vi "ziGetEventPWAWave.vi"(8 "Error In":errorcluster, 10 "PWAWaves In":T1[](array[typedef]) {"Frequency (Hz)" format="%#_6p"}, 11 "Handle In":T2 {"Handle" format="0x%08x"; "Conn" format="0x%08x"}) -> (0 "Error Out":errorcluster, 2 "PWAWaves Out":T1[](array[typedef]) {"Frequency (Hz)" format="%#_6p"}, 3 "Handle Out":T2 {"Handle" format="0x%08x"; "Conn" format="0x%08x"})   [LabVIEW 2009, in "Zurich Instruments LabOne.lvlib"]
uses:
  <instrlib>/Zurich Instruments LabOne/Zurich Instruments LabOne.lvlib
  <instrlib>/Zurich Instruments LabOne/Public/ziTypeHandle.ctl
  <instrlib>/Zurich Instruments LabOne/Public/Data/ziTypePWAWave.ctl
  <instrlib>/Zurich Instruments LabOne/Private/ziLV64.dll
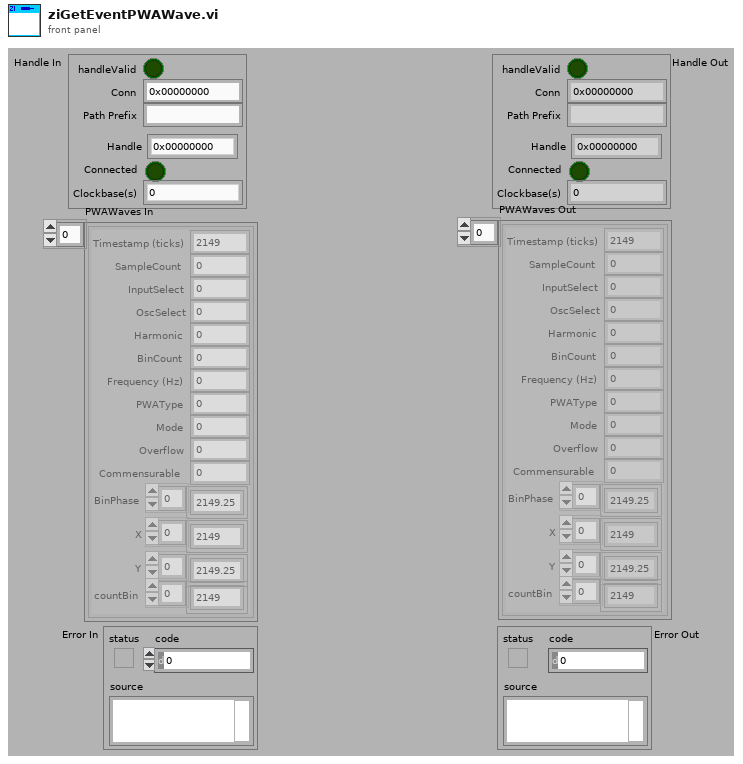
[diagram p1: front panel]
types:
  T1 = typedef "Zurich Instruments LabOne.lvlib/ziTypePWAWave.ctl" = cluster{"Timestamp (ticks)":u64, "SampleCount":u64, "InputSelect":i32, "OscSelect":i32, "Harmonic":i32, "BinCount":i32, "Frequency (Hz)":dbl, "PWAType":u8, "Mode":u8, "Overflow":u8, "Commensurable":u8, "BinPhase":dbl[], "X":dbl[], "Y":dbl[], "countBin":u32[]}
  T2 = typedef "Zurich Instruments LabOne.lvlib/ziTypeHandle.ctl" = cluster{"handleValid":bool, "Conn":u64, "Path Prefix":string, "Handle":u64, "Connected":bool, "Clockbase(s)":dbl}
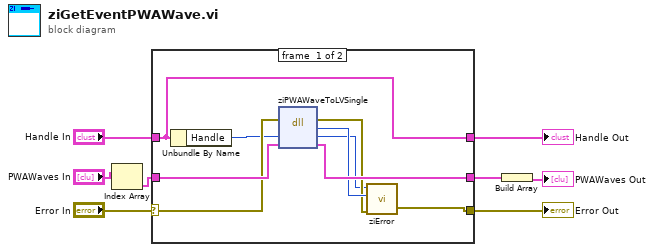
[diagram p0: block diagram]
diagram:
  n1 = Index Array(array="PWAWaves In") -> (element=w2:T1)  [unwired: 1 in]
  n2 = case shown="No Error" "Error In" {
    selector: "Error In" -> [w14 w18]
    tunnel: "Handle In" -> [w10 w20]
    tunnel: [w10 w20] -> w7
    tunnel: [w17 w18] -> w6
    tunnel: w2 -> [w16 w19]
    tunnel: [w15 w19] -> w4
    frame #0 {
      n3 = Unbundle By Name(w10) -> ("Handle"=w13:u64)
      n4 = dll-call lib="C:/Program Files/National Instruments/LabVIEW 2009/instr.lib/Zurich Instruments LabOne/Private/ziLV*.*" fn="ziPWAWaveToLVSingle"(error in=w14, "ziEventBuffer"=w13, "PWAWave"=w16) -> (error out=w11:errorcluster, "return type"=w12:u32, "ziEventBuffer"=w9:u64, "PWAWave"=w15:T1)  [unwired: 2 in, 1 out]
      n5 = call <instrlib>:"ziError.vi"("Conn"=w9, "ziErrorCode"=w12, "Error In"=w11) -> ("Error Out"=w17:errorcluster)  [unwired: 2 in, 1 out]
    }
    frame #1 {
    }
  }
  "Handle Out" <- w7
  "Error Out" <- w6
  n6 = Build Array(w4) -> (→"PWAWaves Out":T1[])
